vi "Filter device group devices.vi"(10 "Device groups to get":string[](array[string]), 11 "device groups all info":string[][](array[string])) -> (3 "Devices":string[](array[string]))   [LabVIEW 2020]
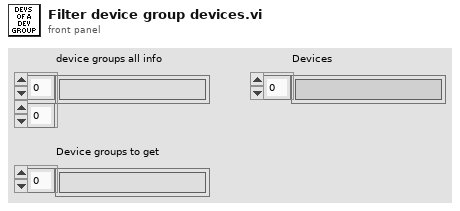
[diagram p1: front panel]
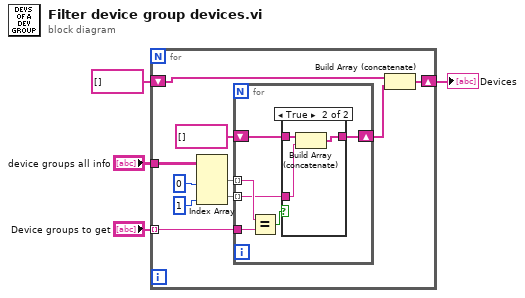
[diagram p0: block diagram]
diagram:
  n1 = for {
    tunnel: "device groups all info" -> [w14]
    tunnel: "Device groups to get" -> [w8] mode=indexing
    shift-right: [w5] -> w3
    shift-left: string[] [] -> [w7]
    n2 = Index Array(array=w14, index (col) #1=0 ("disabled index (col)"), index (col) #2=1 ("index (col)")) -> (element #1=w11:string[], element #2=w10:string[])  [unwired: 2 in]
    n3 = for {
      tunnel: w11 -> [w20] mode=indexing
      tunnel: w8 -> [w19]
      tunnel: w10 -> [w17] mode=indexing
      shift-right: [w16] -> w6
      shift-left: string[] [] -> [w15]
      n4 = Equal?(x=w20, y=w19) -> (x = y?=w18:bool)
      n5 = case shown="True" w18 {
        tunnel: w17 -> [_ w24]
        tunnel: [w21 w23] -> w16
        tunnel: w15 -> [w21 w22]
        frame False {
        }
        frame True {
          n6 = Build Array (concatenate)(w22, w24) -> (w23:string[])
        }
      }
    }
    n7 = Build Array (concatenate)(w7, w6) -> (w5:string[])
  }
  "Devices" <- w3
